vi "GetUnits.vi"(10 "kParNum":i32, 11 "dvotAFTKinetics":refnum<class "dvotAFTKinetics.lvclass">) -> (2 "String":string, 3 "dvotAFTKinetics":refnum<class "dvotAFTKinetics.lvclass">)   [LabVIEW 2012, in "dvotAFTKinetics.lvclass"]
uses:
  dvotAFTKinetics.lvclass
  Constants/dvotAFTConstants.vi
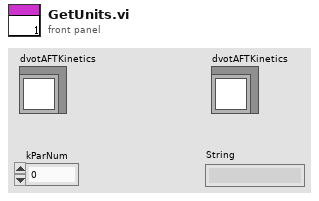
[diagram p1: front panel]
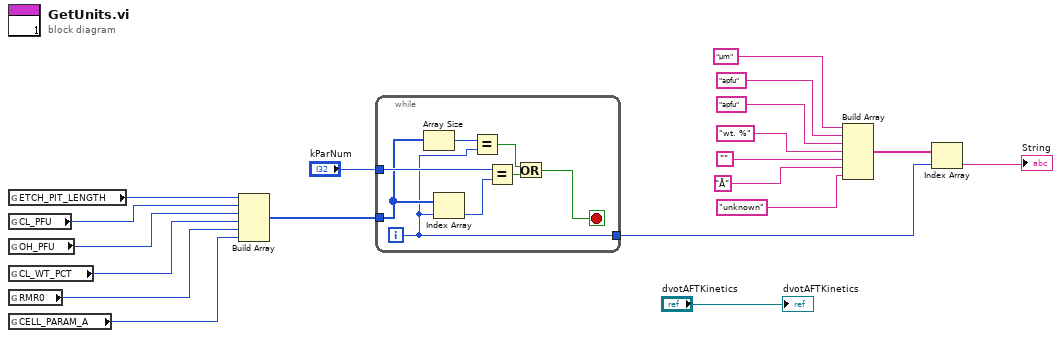
[diagram p0: block diagram]
diagram:
  n1 = global read "dvotAFTConstants.vi" "ETCH_PIT_LENGTH"() -> (w19:i32)
  n2 = global read "dvotAFTConstants.vi" "CL_PFU"() -> (w18:i32)
  n3 = global read "dvotAFTConstants.vi" "OH_PFU"() -> (w17:i32)
  n4 = global read "dvotAFTConstants.vi" "CL_WT_PCT"() -> (w16:i32)
  n5 = global read "dvotAFTConstants.vi" "RMR0"() -> (w15:i32)
  n6 = global read "dvotAFTConstants.vi" "CELL_PARAM_A"() -> (w14:i32)
  n7 = Build Array(w19, w18, w17, w16, w15, w14) -> (w13:i32[])
  n8 = while {
    tunnel: "kParNum" -> [w27]
    tunnel: w13 -> [w26]
    tunnel: [w20] -> w12
    i -> [w20]
    stop <- w21 stop-if-true
    n9 = Array Size(array=w26) -> (size(s)=w25:i32)
    n10 = Index Array(array=w26, index=w20) -> (element=w24:i32)
    n11 = Equal?(x=w25, y=w20) -> (x = y?=w23:bool)
    n12 = Equal?(x=w27, y=w24) -> (x = y?=w22:bool)
    n13 = Or(x=w23, y=w22) -> (x .or. y?=w21:bool)
  }
  n14 = Build Array("µm", "apfu", "apfu", "wt. %", "", "Å", "unknown") -> (w11:string[])
  n15 = Index Array(array=w11, index=w12) -> (element=→"String":string)
  "dvotAFTKinetics" <- "dvotAFTKinetics"
